vi "Version Update.vi"(8 "error in (no error)":errorcluster, 10 "Version":cluster{i32, i32, i32}, 11 "Device Item Ref In in":T1 format="%.0x") -> (0 "error out":errorcluster, 3 "Device Item Ref In out":T1 format="%.0x")   [LabVIEW 2023, in "Vires VTD System Explorer.lvlib"]
uses:
  Vires VTD System Explorer.lvlib
  <vilib>/NI VeriStand/Custom Device API/Custom Device Item Ref.ctl
  Shared/Network Settings_V1.0.x.ctl
  Shared/Protocol.ctl
  Shared/Network Settings.ctl
  Shared/Constants.vi
  <vilib>/NI VeriStand/Custom Device Tools/Custom Device Utility Library/NI VeriStand - Search for Item by Name.vi
  <vilib>/NI VeriStand/Custom Device API/Get Item Property (Variant).vi
  <vilib>/NI VeriStand/Custom Device Tools/Custom Device Utility Library/NI VeriStand - Search for Item by GUID.vi
  <vilib>/NI VeriStand/Custom Device API/Get Item Property (String Array).vi
  <vilib>/NI VeriStand/Custom Device API/Set Item Property (String Array).vi
  Shared/Vires VTD Shared.lvlib
  <vilib>/NI VeriStand/Custom Device API/Custom Device API.lvlib
  <vilib>/NI VeriStand/Custom Device Tools/Custom Device Utility Library/Custom Device Utility Library.lvlib
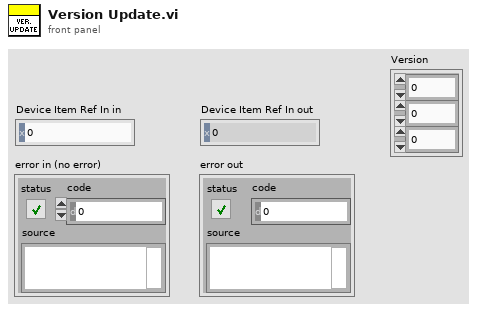
[diagram p1: front panel]
types:
  T1 = typedef "Custom Device API.lvlib/Custom Device Item Ref.ctl" = u64
  T2 = typedef "Vires VTD Shared.lvlib/Protocol.ctl" = enum16{"UDP", "TCP"}
  T3 = typedef "Vires VTD Shared.lvlib/Network Settings.ctl" = cluster{"IP adress":string, "RDB":cluster{"Protocol":T2, "Tx Port":u16, "Rx Port":u16, "Buffer Size":i32, "Timeout":u16}, "SCP":cluster{"Protocol":T2, "Tx Port":u16, "Rx Port":u16, "Buffer Size":i32, "Timeout":u16}}
  T4 = typedef "Vires VTD Shared.lvlib/Network Settings_V1.0.x.ctl" = cluster{"Protocol":T2, "Net Adress":string, "Network Port":u16, "Buffer Size (bytes)":i32, "Timeout (ms)":u16}
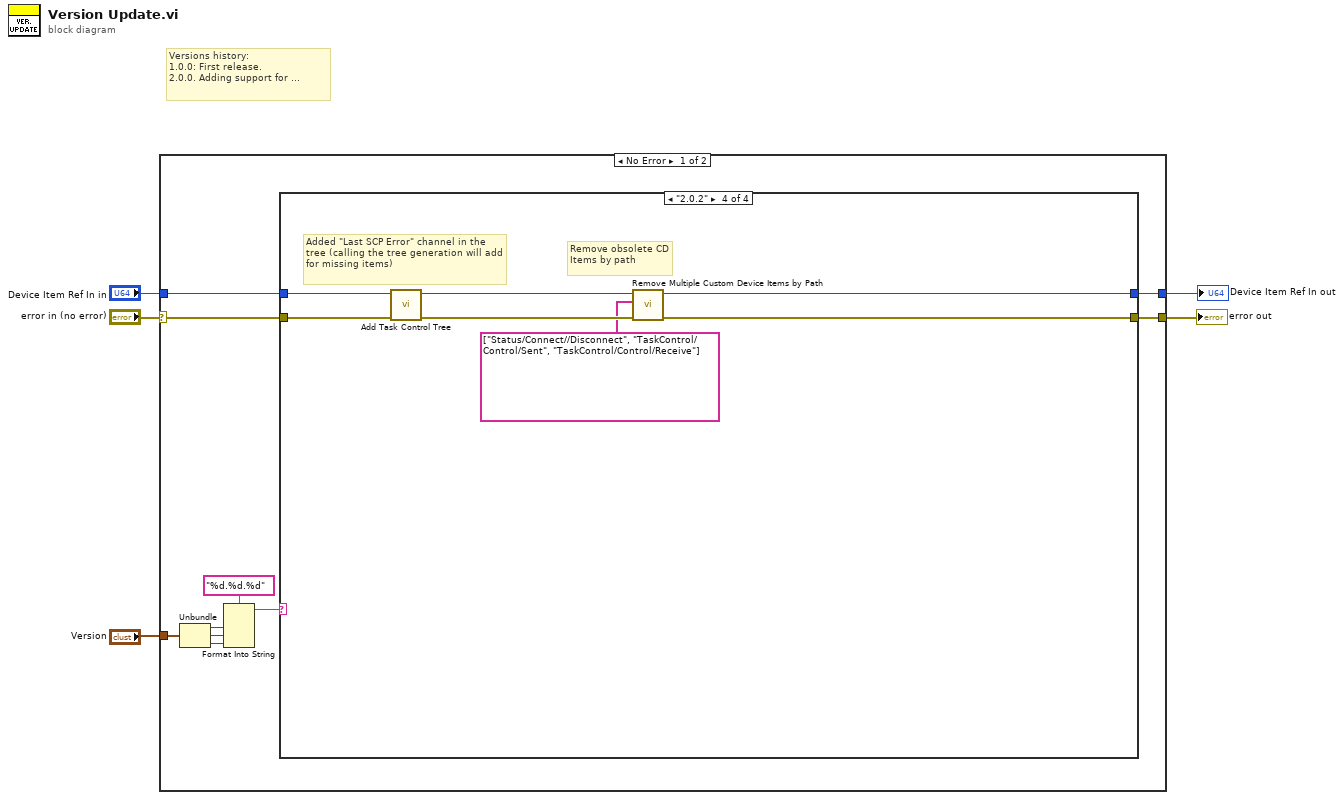
[diagram p0: block diagram]
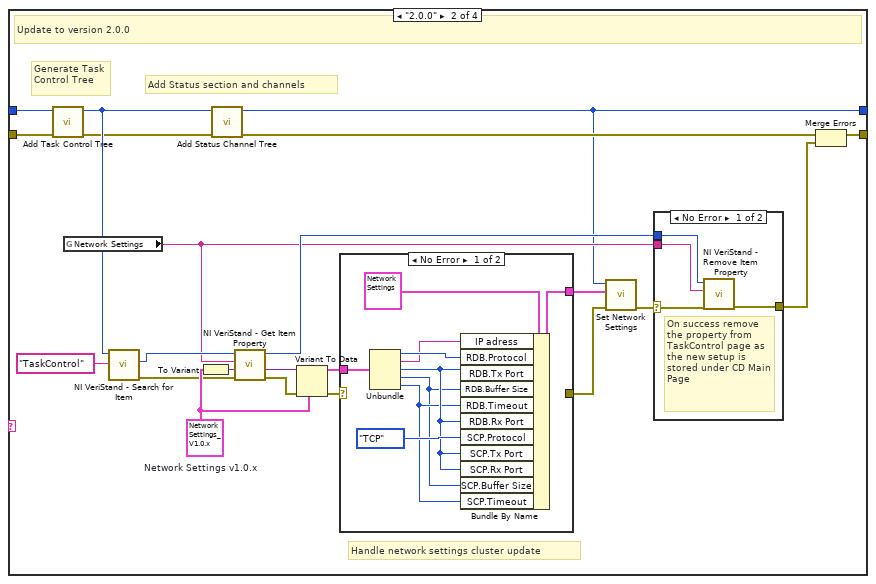
[diagram p3: hidden frame]
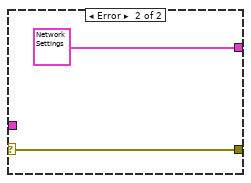
[diagram p4: hidden frame]
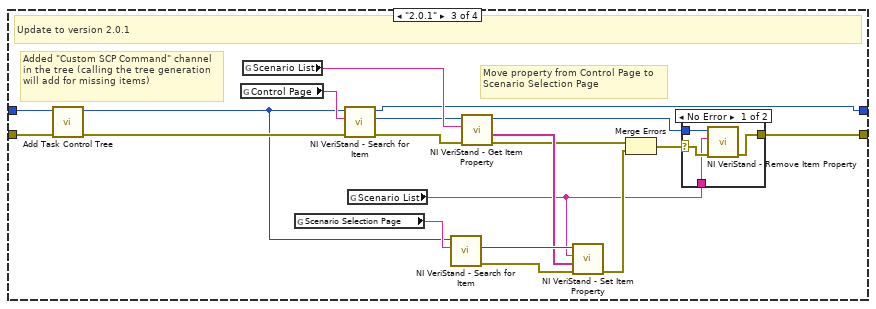
[diagram p6: hidden frame]
diagram:
  # "Versions history:\n1.0.0: First release.\n2.0.0. Adding support for ..."
  n1 = case shown="No Error" "error in (no error)" {
    selector: "error in (no error)" -> [w13 w87]
    tunnel: "Device Item Ref In in" -> [w14 w88]
    tunnel: [w15 w88] -> w3
    tunnel: [w12 w87] -> w2
    tunnel: "Version" -> [w11 _]
    frame No Error {
      n2 = Unbundle(w11) -> (w10:i32, w9:i32, w8:i32)
      n3 = Format Into String(format string="%d.%d.%d", w10, w9, w8) -> (resulting string=w6:string)  [unwired: 2 in, 1 out]
      n4 = case shown="\"2.0.2\"" w6 {
        tunnel: [w17 w22 w65 w83] -> w15
        tunnel: w14 -> [w17 w21 w74 w85]
        tunnel: w13 -> [w16 w19 w73 w86]
        tunnel: [w16 w38 w57 w81] -> w12
        frame Default {
        }
        frame "2.0.0" {
          w33 = T4 {"Protocol"=enum."TCP", "Net Adress"="127.0.0.1", "Network Port"=48190, "Buffer Size (bytes)"=200480, "Timeout (ms)"=10}  # Network Settings v1.0.x
          # "Generate Task Control Tree"
          # "Handle network settings cluster update"
          # "Add Status section and channels"
          # "Update to version 2.0.0"
          n5 = call "Add Task Control Tree.vi"("error in (no error)"=w19, "Item Ref in"=w21) -> ("error out"=w18:errorcluster, "Parent Ref out"=w20:T1)  [unwired: 8 in]
          n6 = global read "Constants.vi" "Network Settings"() -> (w27:string)
          n7 = call-poly <vilib>:"NI VeriStand - Search for Item.vi"("Item Name"="TaskControl", "Section Ref in"=w20) -> ("error out"=w30:errorcluster, "Item Ref"=w29:T1)  [unwired: 6 in, 2 out]
          n8 = To Variant(anything=w33) -> (Variant=w37:variant)
          n9 = call "Add Status Channel Tree.vi"("error in (no error)"=w18, "Parent Ref in"=w20) -> ("error out"=w39:errorcluster, "Parent Ref out"=w22:T1)  [unwired: 8 in]
          n10 = call-poly <vilib>:"NI VeriStand - Get Item Property.vi"("error in (no error)"=w30, "Default Value"=w37, "Property Name"=w27, "Item Ref in"=w29) -> ("error out"=w35:errorcluster, "Value"=w36:variant, "Item Ref out"=w28:T1)  [unwired: 4 in, 1 out]
          n11 = Variant To Data(error in=w35, type=w33, Variant=w36) -> (data=w34:T4, error out=w32:errorcluster)
          n12 = case shown="No Error" w32 {
            selector: w32 -> [_ w50]
            tunnel: w34 -> [w48 _]
            tunnel: [w46 T3 {"IP adress"="127.0.0.1", "RDB"={"Protocol"=enum."TCP", "Tx Port"=48190, "Rx Port"=8192, "Buffer Size"=48190, "Timeout"=10}, "SCP"={"Protocol"=enum."TCP", "Tx Port"=48191, "Rx Port"=8192, "Buffer Size"=48190, "Timeout"=10}} ("Network Settings")] -> w25
            tunnel: [_ w50] -> w24
            frame No Error {
              n13 = Unbundle(w48) -> ("Protocol"=w45:T2, "Net Adress"=w44:string, "Network Port"=w42:u16, "Buffer Size (bytes)"=w40:i32, "Timeout (ms)"=w41:u16)
              n14 = Bundle By Name(cluster=T3 {"IP adress"="127.0.0.1", "RDB"={"Protocol"=enum."TCP", "Tx Port"=48190, "Rx Port"=8192, "Buffer Size"=48190, "Timeout"=10}, "SCP"={"Protocol"=enum."TCP", "Tx Port"=48191, "Rx Port"=8192, "Buffer Size"=48190, "Timeout"=10}} ("Network Settings"), "IP adress"=w44, "RDB.Protocol"=w45, "RDB.Tx Port"=w42, "RDB.Buffer Size"=w40, "RDB.Timeout"=w41, "RDB.Rx Port"=w42, "SCP.Protocol"=Protocol."TCP", "SCP.Tx Port"=w42, "SCP.Rx Port"=w42, "SCP.Buffer Size"=w40, "SCP.Timeout"=w41) -> (w46:T3)
            }
            frame Error {
            }
          }
          n15 = call "Set Network Settings.vi"("error in"=w24, "Network Settings"=w25, "Item Ref in"=w22) -> ("error out"=w23:errorcluster)  [unwired: 7 in, 1 out]
          n16 = case shown="No Error" w23 {
            selector: w23 -> [w54 w55]
            tunnel: w28 -> [w53 _]
            tunnel: w27 -> [w52 _]
            tunnel: [w51 w55] -> w26
            frame No Error {
              # "On success remove the property from TaskControl page as the new setup is stored under CD Main Page"
              n17 = call <vilib>:"NI VeriStand - Remove Item Property.vi"("error in (no error)"=w54, "Property Name"=w52, "Item Ref in"=w53) -> ("error out"=w51:errorcluster)  [unwired: 6 in, 2 out]
            }
            frame Error {
              # "Let process to generate error"
            }
          }
          n18 = Merge Errors(w39, w26) -> (w38:errorcluster)
        }
        frame "2.0.1" {
          # "Move property from Control Page to Scenario Selection Page"
          # "Added \"Custom SCP Command\" channel in the tree (calling the tree generation will add for missing items)"
          # "Update to version 2.0.1"
          n19 = call "Add Task Control Tree.vi"("error in (no error)"=w73, "Item Ref in"=w74) -> ("error out"=w68:errorcluster, "Parent Ref out"=w66:T1)  [unwired: 8 in]
          n20 = global read "Constants.vi" "Control Page"() -> (w72:string)
          n21 = global read "Constants.vi" "Scenario List"() -> (w71:string)
          n22 = global read "Constants.vi" "Scenario Selection Page"() -> (w67:string)
          n23 = call-poly <vilib>:"NI VeriStand - Search for Item.vi"("error in"=w68, "Item GUID"=w72, "Section Ref in"=w66) -> ("error out"=w70:errorcluster, "Item Ref"=w69:T1, "Section Ref out"=w65:T1)  [unwired: 5 in, 1 out]
          n24 = global read "Constants.vi" "Scenario List"() -> (w56:string)
          n25 = call-poly <vilib>:"NI VeriStand - Search for Item.vi"("Item GUID"=w67, "Section Ref in"=w66) -> ("error out"=w63:errorcluster, "Item Ref"=w64:T1)  [unwired: 6 in, 2 out]
          n26 = call-poly <vilib>:"NI VeriStand - Get Item Property.vi"("error in (no error)"=w70, "Property Name"=w71, "Item Ref in"=w69) -> ("error out"=w61:errorcluster, "Value"=w62:string[], "Item Ref out"=w60:T1)  [unwired: 5 in, 1 out]
          n27 = call-poly <vilib>:"NI VeriStand - Set Item Property.vi"("error in (no error)"=w63, "Value"=w62, "Property Name"=w56, "Item Ref in"=w64) -> ("error out"=w59:errorcluster)  [unwired: 5 in, 2 out]
          n28 = Merge Errors(w61, w59) -> (w58:errorcluster)
          n29 = case shown="No Error" w58 {
            selector: w58 -> [w77 w79]
            tunnel: w60 -> [w78 _]
            tunnel: [w76 w79] -> w57
            tunnel: w56 -> [w75 _]
            frame No Error {
              n30 = call <vilib>:"NI VeriStand - Remove Item Property.vi"("error in (no error)"=w77, "Property Name"=w75, "Item Ref in"=w78) -> ("error out"=w76:errorcluster)  [unwired: 6 in, 2 out]
            }
            frame Error {
            }
          }
        }
        frame "2.0.2" {
          # "Remove obsolete CD Items by path"
          # "Added \"Last SCP Error\" channel in the tree (calling the tree generation will add for missing items)"
          n31 = call "Add Task Control Tree.vi"("error in (no error)"=w86, "Item Ref in"=w85) -> ("error out"=w82:errorcluster, "Parent Ref out"=w84:T1)  [unwired: 8 in]
          n32 = call "Remove Multiple Custom Device Items by Path.vi"("error in"=w82, "Paths of Items to Remove"=string[] ["Status/Connect//Disconnect", "TaskControl/Control/Sent", "TaskControl/Control/Receive"], "Device Item Ref in"=w84) -> ("error out"=w81:errorcluster, "Device Item Ref out"=w83:T1)  [unwired: 7 in]
        }
      }
    }
    frame Error {
    }
  }
  "error out" <- w2
  "Device Item Ref In out" <- w3
